vi "Extract Image Header.vi"(8 "error in (no error)":errorcluster, 11 "Queue in":refnum<queue>) -> (0 "error out":errorcluster, 2 "image header":string, 3 "Queue out":refnum<queue>)   [LabVIEW 2013]
uses:
  <vilib>/regexp/Match Regular Expression.xnode
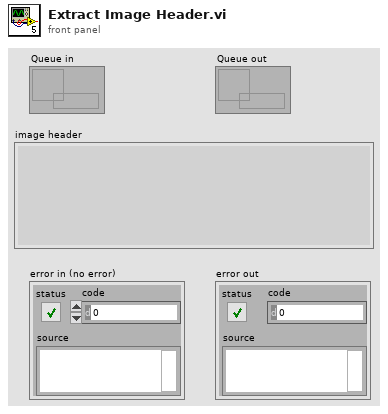
[diagram p1: front panel]
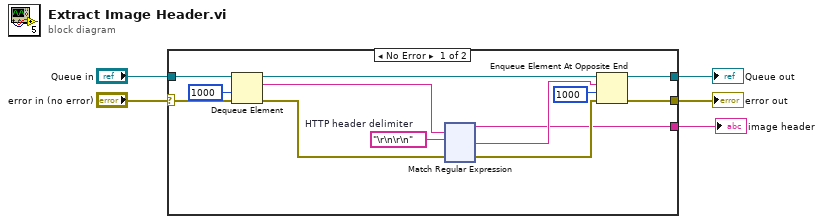
[diagram p0: block diagram]
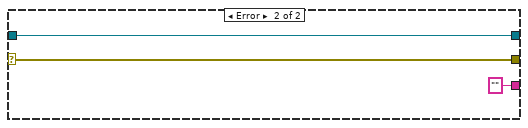
[diagram p2: hidden frame]
diagram:
  n1 = case shown="No Error" "error in (no error)" {
    selector: "error in (no error)" -> [w6 w135]
    tunnel: [w18 w135] -> w5
    tunnel: [w15 w134] -> w4
    tunnel: [w10 "" ("before match")] -> w3
    tunnel: "Queue in" -> [w7 w134]
    frame No Error {
      w9 = "\r\n\r\n"  # HTTP header delimiter
      n2 = Dequeue Element(queue=w7, timeout in ms (-1)=1000, error in (no error)=w6) -> (queue out=w13:refnum<queue>, element=w11:string, error out=w16:errorcluster)  [unwired: 1 out]
      n3 = xnode "Match Regular Expression"("input string"=w11, "regular expression"=w9, "error in"=w16) -> ("before match"=w10:string, "after match"=w14:string, "error out"=w17:errorcluster)  [unwired: 3 in, 2 out]
      n4 = Enqueue Element At Opposite End(queue=w13, element=w14, timeout in ms (-1)=1000, error in (no error)=w17) -> (queue out=w15:refnum<queue>, error out=w18:errorcluster)  [unwired: 1 out]
    }
    frame Error {
    }
  }
  "image header" <- w3
  "error out" <- w5
  "Queue out" <- w4
